vi "Pre Launch Init.vi"(11 "AirMar150WX in":refnum<class "AirMar150WX.lvclass">) -> (0 "error out":errorcluster, 3 "AirMar150WX out":refnum<class "AirMar150WX.lvclass">)   [LabVIEW 2017, in "AirMar 150WX.lvlib" / "AirMar150WX.lvclass"]
doc: "Sends a high priority message to it's self to notify the monitor that it's spawned. If it's in the runtime environment, this message is never sent, meaning the monitor will never spawn\n\nCopyright: MGI\nAuthored by: Derek Trepanier"
uses:
  AirMar150WX.lvclass
  AirMar150WX.lvclass/AirMar150WX.ctl
  Sensor Actor/Sensor/Sensor.lvclass
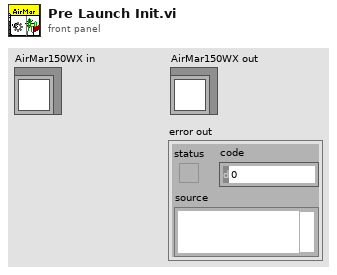
[diagram p1: front panel]
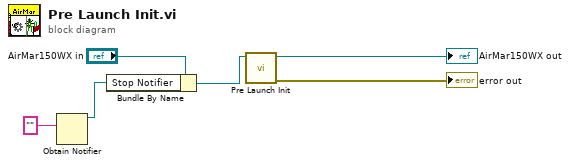
[diagram p0: block diagram]
diagram:
  n1 = Obtain Notifier(notification data type="" ("name (unnamed)")) -> (notifier out=w3:refnum<notifier>)  [unwired: 3 in, 2 out]
  n2 = Bundle By Name(cluster="AirMar150WX in", "Stop Notifier"=w3) -> (w1:refnum<class "AirMar150WX.lvclass">)
  n3 = call-parent "Pre Launch Init.vi"("Sensor in"=w1) -> ("error out"=→"error out":errorcluster, "Sensor out"=→"AirMar150WX out":refnum<class "AirMar150WX.lvclass">)  [unwired: 9 in]
